vi "helper1.vi"(8 "error in (no error)":errorcluster, 11 "y":string="Sub Panel") -> (0 "error out":errorcluster, 3 "Array":string[](array[string]))   [LabVIEW 2016]
panel:
  out "Array 2":string[](array[string])
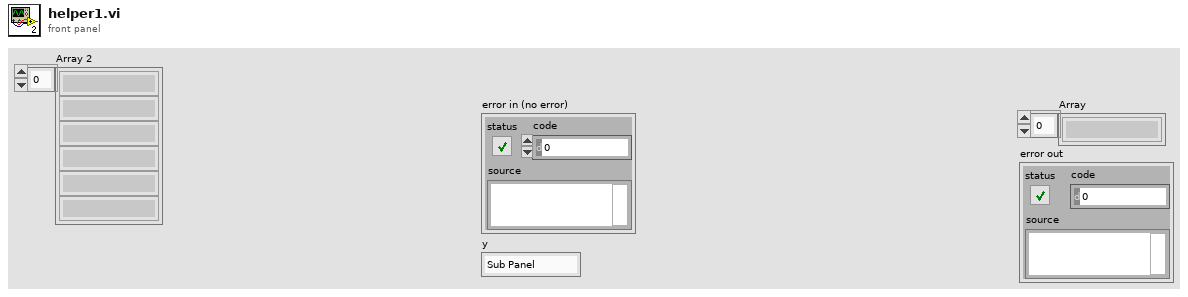
[diagram p1: front panel]
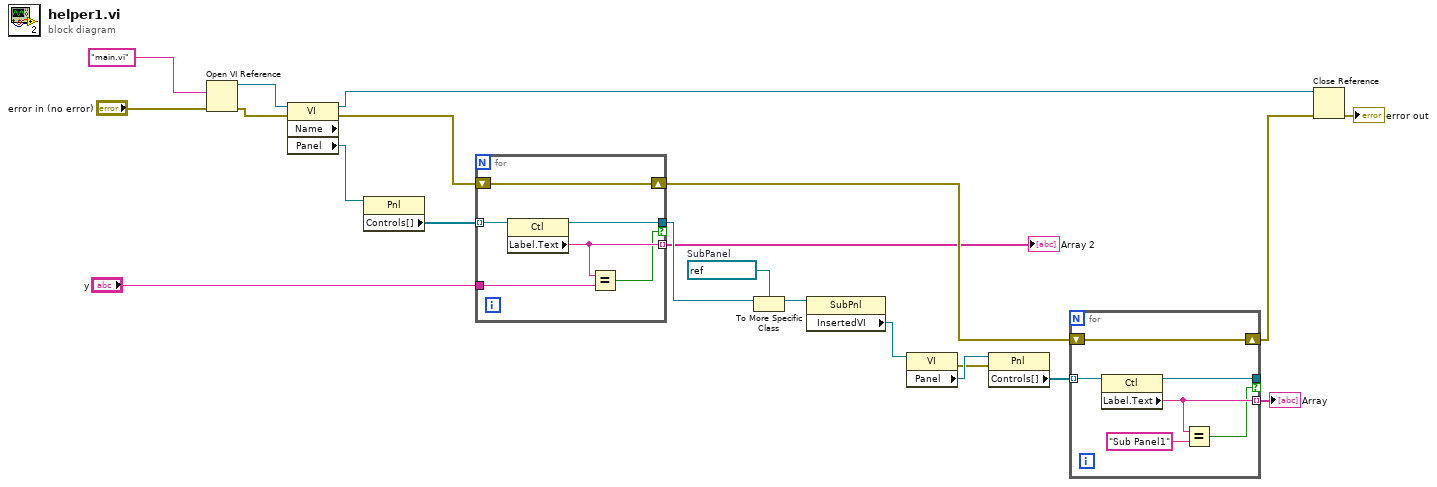
[diagram p0: block diagram]
diagram:
  w15 = refnum<vi> refnum  # SubPanel
  n1 = Open VI Reference(vi path="main.vi" ("machine name (\"\":  open local reference)"), error in (no error)="error in (no error)") -> (vi reference=w7:refnum<vi>, error out=w6:errorcluster)  [unwired: 4 in]
  n2 = property class="VI" props=["Name", "Panel"](reference=w7, error in=w6) -> (reference out=w8:refnum<vi>, error out=w12:errorcluster, "Panel"=w9:refnum<vi>)  [unwired: 1 out]
  n3 = property class="Pnl"(reference=w9) -> ("Controls[]"=w10:refnum<vi>[])  [unwired: 1 in, 2 out]
  n4 = for {
    tunnel: w10 -> [w27] mode=indexing
    tunnel: [w25] -> w11 mode=indexing
    shift-right: [w26] -> w17
    shift-left: w12 -> [w26]
    tunnel: [w24] -> w13 if=w23
    tunnel: "y" -> [w22]
    n5 = property class="Ctl"(reference=w27) -> (reference out=w24:refnum<vi>, "Label.Text"=w25:string)  [unwired: 1 in, 1 out]
    n6 = Equal?(x=w25, y=w22) -> (x = y?=w23:bool)
  }
  "Array 2" <- w11
  n7 = To More Specific Class(target class=w15, reference=w13) -> (specific class reference=w14:refnum<vi>)  [unwired: 1 in, 1 out]
  n8 = property class="SubPnl"(reference=w14) -> ("InsertedVI"=w20:refnum<vi>)  [unwired: 1 in, 2 out]
  n9 = property class="VI"(reference=w20) -> (error out=w19:errorcluster, "Panel"=w21:refnum<vi>)  [unwired: 1 in, 1 out]
  n10 = property class="Pnl"(reference=w21, error in=w19) -> ("Controls[]"=w16:refnum<vi>[])  [unwired: 2 out]
  n11 = for {
    tunnel: w16 -> [w33] mode=indexing
    tunnel: [w31] -> w3 mode=indexing
    shift-right: [w32] -> w18
    shift-left: w17 -> [w32]
    tunnel: [w29] -> _ if=w28
    n12 = property class="Ctl"(reference=w33) -> (reference out=w29:refnum<vi>, "Label.Text"=w31:string)  [unwired: 1 in, 1 out]
    n13 = Equal?(x=w31, y="Sub Panel1") -> (x = y?=w28:bool)
  }
  "Array" <- w3
  n14 = Close Reference(reference=w8, error in (no error)=w18) -> (error out=→"error out":errorcluster)
